vi "MouseSim.vi"() -> ()   [LabVIEW 2016]
uses:
  Source/main/apis/Setup/GetControlRef/GetControlRefByPath.vi
  User32.dll
  Source/main/apis/Setup/GetControlRef/GetControlRef.lvlib
panel:
  in  "error in":errorcluster
  out "error out":errorcluster
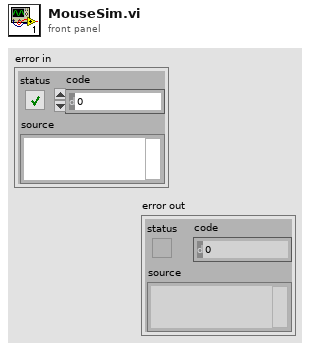
[diagram p1: front panel]
types:
  T1 = typedef "LVRectTypeDef.ctl" = cluster{"Left":i16, "Top":i16, "Right":i16, "Bottom":i16}
  T2 = typedef "LVPositionTypeDef.ctl" = cluster{"Left":i32, "Top":i32}
  T3 = typedef "LVPointTypeDef.ctl" = cluster{"Horizontal":i16, "Vertical":i16}
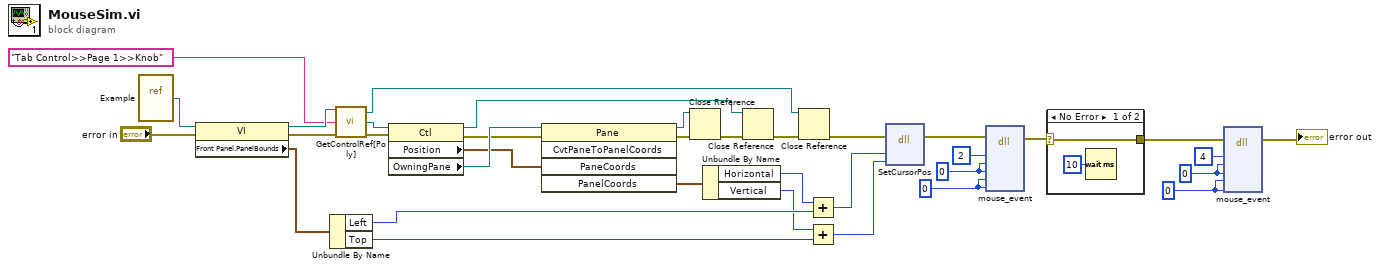
[diagram p0: block diagram]
diagram:
  w33 = 0 ("dwExtraInfo")
  w34 = u32 0 ("dwExtraInfo")
  w32 = 0 ("dwExtraInfo")
  w31 = u32 0 ("dwExtraInfo")
  n1 = vi-ref "Example.vi"() -> (w20:refnum<vi>)
  n2 = property class="VI"(reference=w20, error in="error in") -> (reference out=w22:refnum<vi>, error out=w24:errorcluster, "Front Panel.PanelBounds"=w19:T1)
  n3 = Unbundle By Name(w19) -> ("Left"=w17:i16, "Top"=w15:i16)
  n4 = call-poly "GetControlRef[Poly].vi"("VI Reference In"=w22, "Control Path"="Tab Control>>Page 1>>Knob", "error In"=w24) -> ("VI Reference Out"=w1:refnum<vi>, "Ctl Refnum"=w23:refnum<vi>, "error out"=w25:errorcluster)  [unwired: 10 in]
  n5 = property class="Ctl"(reference=w23, error in=w25) -> (reference out=w3:refnum<vi>, error out=w9:errorcluster, "Position"=w11:T2, "OwningPane"=w12:refnum<vi>)
  n6 = invoke class="Pane" method="CvtPaneToPanelCoords"(reference=w12, error in=w9, "PaneCoords"=w11) -> (reference out=w5:refnum<vi>, error out=w8:errorcluster, "PanelCoords"=w10:T3)  [unwired: 2 in, 2 out]
  n7 = Close Reference(reference=w5, error in (no error)=w8) -> (error out=w6:errorcluster)
  n8 = Unbundle By Name(w10) -> ("Horizontal"=w18:i16, "Vertical"=w16:i16)
  n9 = Close Reference(reference=w3, error in (no error)=w6) -> (error out=w4:errorcluster)
  n10 = Close Reference(reference=w1, error in (no error)=w4) -> (error out=w2:errorcluster)
  n11 = Add(x=w18, y=w17) -> (x+y=w13:i16)
  n12 = Add(x=w16, y=w15) -> (x+y=w14:i16)
  n13 = dll-call lib="user32.dll" fn="SetCursorPos" label="Move mouse"(error in=w2, "dx"=w13, "dy"=w14) -> (error out=w27:errorcluster)  [unwired: 5 in, 1 out]
  n14 = dll-call lib="user32.dll" fn="mouse_event" label="Click"(error in=w27, "dwFlags"=2, "dx"=w32, "dy"=w32, "dwData"=w31, "dwExtraInfo"=w31) -> (error out=w29:errorcluster)  [unwired: 8 in, 1 out]
  n15 = case shown="No Error" w29 {
    selector: w29 -> [w36 w38]
    tunnel: [w36 w38] -> w28
    frame No Error {
      n16 = Wait (ms)(milliseconds to wait=u32 10) -> ()  [unwired: 1 out]
    }
    frame Error {
    }
  }
  n17 = dll-call lib="user32.dll" fn="mouse_event" label="Release"(error in=w28, "dwFlags"=4, "dx"=w33, "dy"=w33, "dwData"=w34, "dwExtraInfo"=w34) -> (error out=→"error out":errorcluster)  [unwired: 8 in, 1 out]
